vi "mainActivity_打开模块的消息簇.vi"(3 "是否移除前模块":string(combo)="NotRemove", 4 "前面板状态":string(combo)="FP_Insert", 5 "是否等待":string(combo)="false", 6 "模块注册信息":T1) -> (0 "消息簇":cluster{"相对路径":string, string[]})   [LabVIEW 2014]
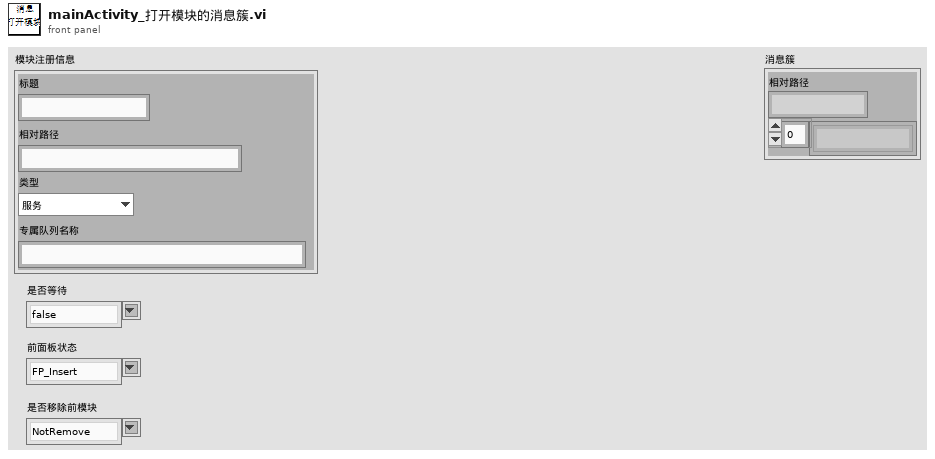
[diagram p1: front panel]
types:
  T1 = cluster{"标题":string, "相对路径":string, "类型":enum16{"服务", "活动"}, "专属队列名称":string}
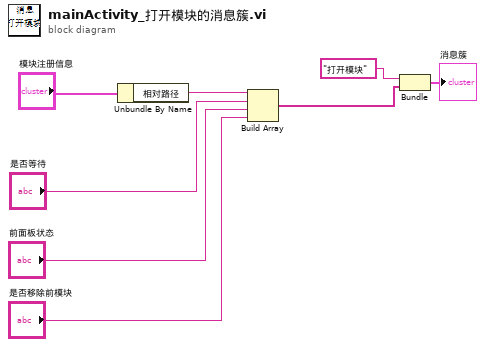
[diagram p0: block diagram]
diagram:
  n1 = Unbundle By Name("模块注册信息") -> ("相对路径"=w7:string)
  n2 = Build Array(w7, "是否等待", "前面板状态", "是否移除前模块") -> (w3:string[])
  n3 = Bundle("相对路径"="打开模块", w3) -> (→"消息簇":cluster{"相对路径":string, string[]})  [unwired: 1 in]
